vi "Drive_Execute.vi"   [LabVIEW 2019]
uses:
  Globals/Drive_Globals.vi
  <vilib>/Rock Robotics/WPI/Joystick/WPI_JoystickArcadeMapping.vi
  <vilib>/Rock Robotics/WPI/ThirdParty/Phoenix-LabVIEW/Motor Controller/Controls/CTRE_Phoenix_MotorControl_ControlMode.ctl
types:
  T1 = typedef "WPI_MotorControlDeviceRef.ctl" = cluster{"DeviceStatus":errorcluster, "Type":T2, "PWM":cluster{"PWM Channel":T3, "DeadBand":T4}, "CAN":cluster{"Device Number":u8, "SetOutput VI Ref":variant, "GetOutput VI Ref":variant, "Enable VI Ref":variant, "Disable VI Ref":variant, "Data":variant}, "Invert":bool, "DIO PWM":cluster{"PWM \"Enable\" Channel":T3, "DIOChannel":T5, "PWM Rate":dbl}}
  T2 = typedef "WPI_MotorControlType.ctl" = enum16{"PWM", "CAN", "DIO PWM"}
  T3 = typedef "FPGA_DIOPWMChannel.ctl" = enum8{"PWM 0", "PWM 1", "PWM 2", "PWM 3", "PWM 4", "PWM 5", "PWM 6", "PWM 7", "PWM 8", "PWM 9", "PWM MXP 0", "PWM MXP 1", "PWM MXP 2", "PWM MXP 3", "PWM MXP 4", "PWM MXP 5", "PWM MXP 6", "PWM MXP 7", "PWM MXP 8", "PWM MXP 9", "Invalid"}
  T4 = typedef "WPI_PWMDeadband.ctl" = cluster{"Name":string, "maxPositivePwm":i32, "minPositivePwm":i32, "centerPwm":i32, "maxNegativePwm":i32, "minNegativePwm":i32, "angularRange":u16}
  T5 = typedef "FPGA_DIOChannel.ctl" = enum8{"DIO 0", "DIO 1", "DIO 2", "DIO 3", "DIO 4", "DIO 5", "DIO 6", "DIO 7", "DIO 8", "DIO 9", "DIO MXP 0", "DIO MXP 1", "DIO MXP 2", "DIO MXP 3", "DIO MXP 4", "DIO MXP 5", "DIO MXP 6", "DIO MXP 7", "DIO MXP 8", "DIO MXP 9", "DIO MXP 10", "DIO MXP 11", "DIO MXP 12", "DIO MXP 13", "DIO MXP 14", "DIO MXP 15", "SPI Port CS1", "SPI Port CS2", "SPI Port CS3", "SPI Port MISO", "SPI Port MOSI", "Invalid"}
  T6 = typedef "Drive_Cluster.ctl" = cluster{"Control_State":T7, "Angular_Throttle":dbl, "Linear_Throttle":dbl, "Torque_Changing":bool}
  T7 = typedef "Drive_States.ctl" = enum16{"Percent_Voltage_Control", "Speed_Control"}
  T8 = typedef "CTRE_Phoenix_MotorControl_ControlMode.ctl" = u16
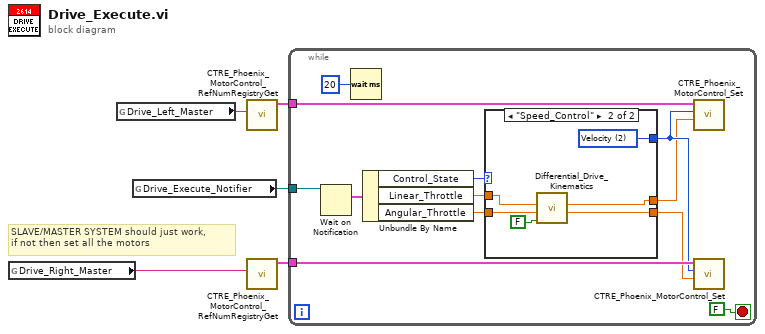
[diagram p0: block diagram]
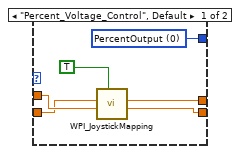
[diagram p2: hidden frame]
diagram:
  # "SLAVE/MASTER SYSTEM should just work, \nif not then set all the motors"
  n1 = global read "Drive_Globals.vi" "Drive_Right_Master"() -> (w3:string)
  n2 = global read "Drive_Globals.vi" "Drive_Left_Master"() -> (w4:string)
  n3 = global read "Drive_Globals.vi" "Drive_Execute_Notifier"() -> (w5:refnum<notifier>)
  n4 = call <vilib>:"CTRE_Phoenix_MotorControl_RefNumRegistryGet.vi"("refnum name"=w4) -> ("PhoenixMotorControlDevRef"=w2:T1)  [unwired: 9 in, 1 out]
  n5 = call <vilib>:"CTRE_Phoenix_MotorControl_RefNumRegistryGet.vi"("refnum name"=w3) -> ("PhoenixMotorControlDevRef"=w1:T1)  [unwired: 9 in, 1 out]
  n6 = while {
    tunnel: w5 -> [w17]
    tunnel: w2 -> [w10]
    tunnel: w1 -> [w9]
    stop <- FALSE stop-if-true
    n7 = Wait on Notification(notifier=w17) -> (notification=w16:T6)  [unwired: 3 in, 3 out]
    n8 = Wait (ms)(milliseconds to wait=u32 20) -> ()  [unwired: 1 out]
    n9 = Unbundle By Name(w16) -> ("Control_State"=w15:T7, "Linear_Throttle"=w13:dbl, "Angular_Throttle"=w12:dbl)
    n10 = case shown="\"Speed_Control\"" w15 {
      tunnel: w13 -> [w23 w28]
      tunnel: w12 -> [w22 w27]
      tunnel: [w21 w26] -> w6
      tunnel: [w20 w25] -> w8
      tunnel: [w18 w24] -> w7
      frame "Percent_Voltage_Control", Default {
        w18 = T8 0 items=["PercentOutput"=0, "Position"=1, "Velocity"=2, "Current"=3, "Follower"=5, "MotionProfile"=6, "MotionMagic"=7, "MotionProfileArc"=10, "Disabled"=15] ("Control Mode")
        n11 = call-poly <vilib>:"WPI_JoystickMapping.vi"("Square Inputs"=TRUE, "Y axis value"=w23, "X axis value"=w22) -> ("Right Motor Value"=w20:dbl, "Left Motor Value"=w21:dbl)  [unwired: 7 in]
      }
      frame "Speed_Control" {
        w24 = T8 2 items=["PercentOutput"=0, "Position"=1, "Velocity"=2, "Current"=3, "Follower"=5, "MotionProfile"=6, "MotionMagic"=7, "MotionProfileArc"=10, "Disabled"=15] ("Control Mode")
        n12 = call "Differential_Drive_Kinematics.vi"("Scale_Down_For_Turn"=FALSE, "Angular_Throttle"=w27, "Linear_Throttle"=w28) -> ("Right_Motor_Velocity"=w25:dbl, "Left_Motor_Velocity"=w26:dbl)  [unwired: 7 in]
      }
    }
    n13 = call <vilib>:"CTRE_Phoenix_MotorControl_Set.vi"("Output"=w6, "Control Mode"=w7, "PhoenixMotorControlDevRef"=w10) -> ()  [unwired: 7 in, 2 out]
    n14 = call <vilib>:"CTRE_Phoenix_MotorControl_Set.vi"("Output"=w8, "Control Mode"=w7, "PhoenixMotorControlDevRef"=w9) -> ()  [unwired: 7 in, 2 out]
  }
